vi "C-ScanPage.vi"() -> ()   [LabVIEW 2026]
panel:
  in  "C Scan Settings":T1
  in  "C-Scan":string(combo)
  out "Axis Controls 3":T2
  in  "E-Stop Reset 3":bool
  out "C-SCAN GRAPH":cluster{"timebase":dbl[], "data":u16[]}[](graph)
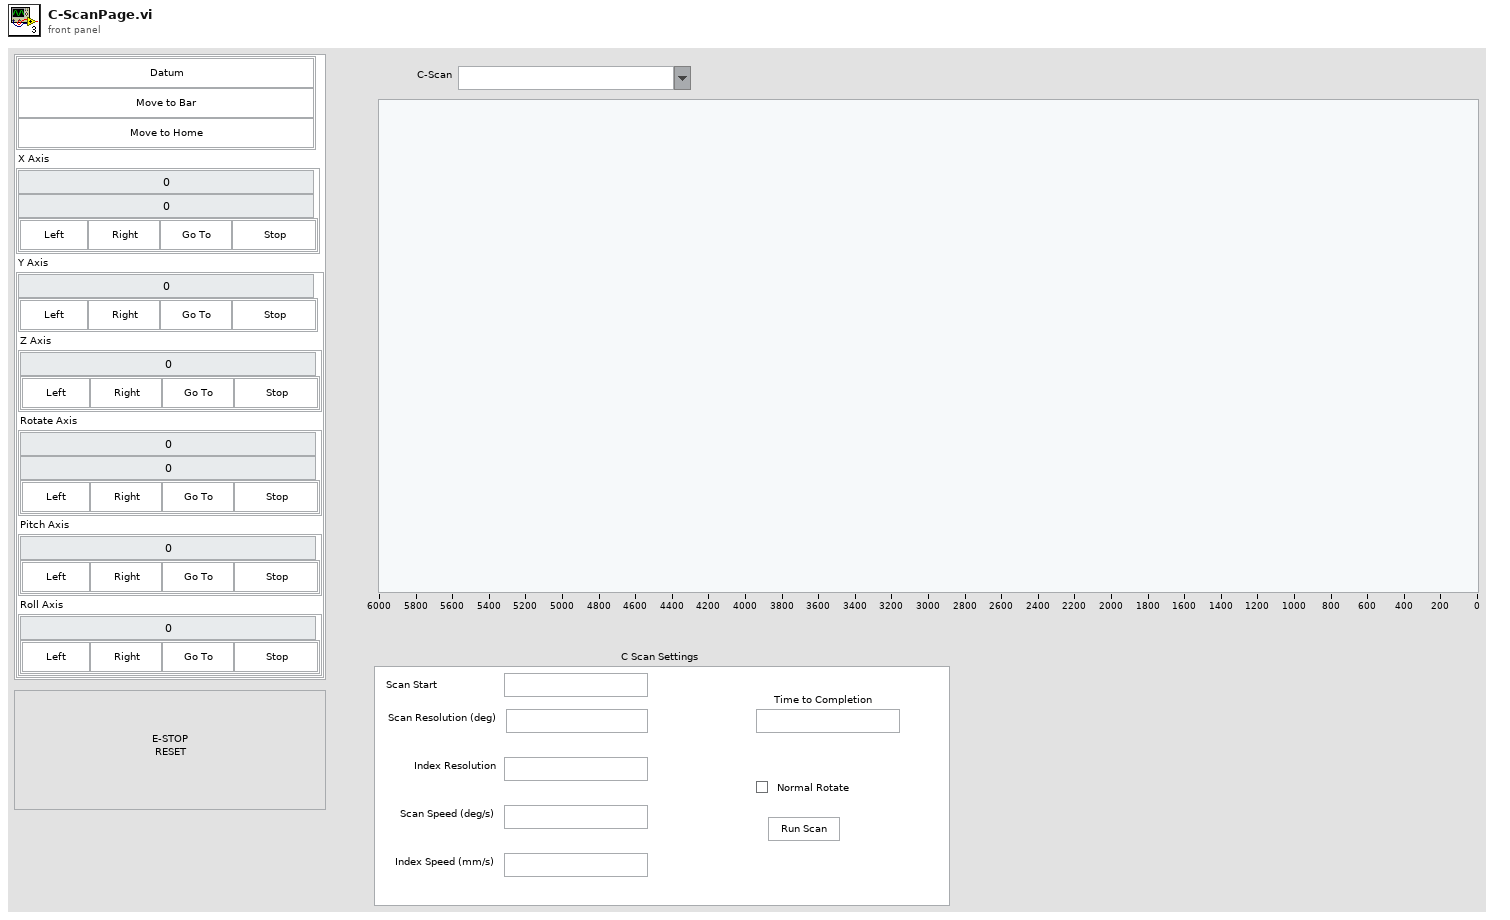
[diagram p1: front panel]
types:
  T1 = cluster{"Scan Start\n":string, "Scan Resolution (deg)\n":string, "Index Resolution":string, "Scan Speed (deg/s)":string, "Index Speed (mm/s)":string, "Time to Completion":string, "Normal Rotate":bool, bool}
  T2 = cluster{"Buttons":cluster{"Datum":bool, "Move to Bar":bool, "Move to Home":bool}, "X Axis":cluster{"Calculated X Value":dbl, "Encoder X Value":dbl, "X Axis Movement Buttons":cluster{"Left":bool, "Right":bool, "Go To":bool, "Stop":bool}}, "Y Axis":cluster{"Encoder Y Value":dbl, "Y Axis Movement Buttons":cluster{"Left":bool, "Right":bool, "Go To":bool, "Stop":bool}, "Z Axis":cluster{"Encoder Z Value":dbl, "Z Axis Movement Buttons":cluster{"Left":bool, "Right":bool, "Go To":bool, "Stop":bool}}, "Rotate Axis":cluster{"Calculated Rotate Value":dbl, "Encoder Rotate Value":dbl, "Rotate Axis Movement Buttons":cluster{"Left":bool, "Right":bool, "Go To":bool, "Stop":bool}}, "Pitch Axis":cluster{"Encoder Pitch Value":dbl, "Pitch Axis Movement Buttons":cluster{"Left":bool, "Right":bool, "Go To":bool, "Stop":bool}}, "Roll Axis":cluster{"Encoder Roll Value":dbl, "Roll Axis Movement Buttons":cluster{"Left":bool, "Right":bool, "Go To":bool, "Stop":bool}}}}
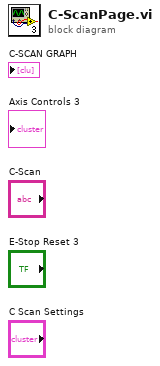
[diagram p0: block diagram]
diagram:
